vi "Read component name.vi"(8 "error in":errorcluster, 11 "DecideProjectFeatures in":refnum<class "DCAFConfigurablePluginDecideFeatures.lvclass">) -> (0 "error out":errorcluster, 2 "component name":string, 3 "DecideProjectFeatures out":refnum<class "DCAFConfigurablePluginDecideFeatures.lvclass">)   [LabVIEW 2013, in "DCAFConfigurablePluginDecideFeatures.lvclass"]
uses:
  DCAFConfigurablePluginDecideFeatures.lvclass
  DCAFConfigurablePluginDecideFeatures.lvclass/DCAFConfigurablePluginDecideFeatures.ctl
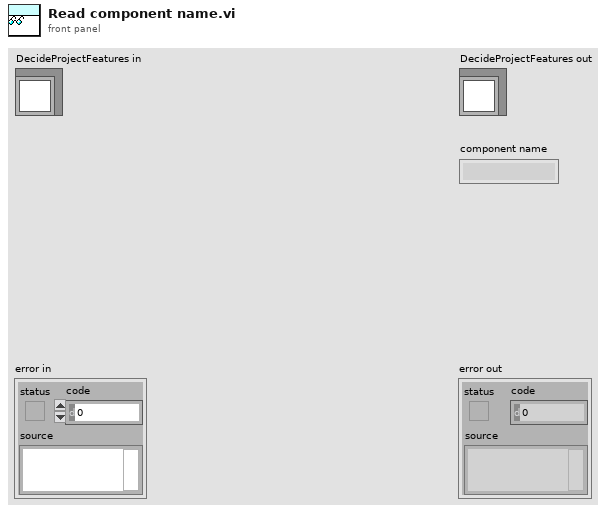
[diagram p1: front panel]
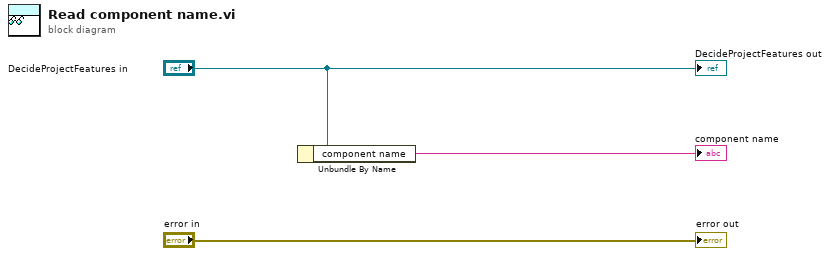
[diagram p0: block diagram]
diagram:
  n1 = Unbundle By Name("DecideProjectFeatures in") -> ("component name"=→"component name":string)
  "error out" <- "error in"
  "DecideProjectFeatures out" <- "DecideProjectFeatures in"
